vi "getPieces.vi"(0 "Refnum in":T1, 5 "Bounding Box":cluster{"x":sgl, "y":sgl}[][](array[cluster]), 7 "Position":sgl[][](array[numeric]), 9 "Angle":sgl[](array[numeric]), 11 "error in (no error)":errorcluster, 12 "Step":sgl=0.29742944, 13 "Origin Pixel":dbl[](array[numeric])) -> (4 "Refnum out":T1, 8 "Data Pieces":T3(array[cluster]) {"ROI Números"."Contours"."Type" items=["No Selection", "Point", "Line", "Rectangle", "Oval", "Polygon", "Freehand Region", "Annulus", "Unused2", "Unused3", "Broken Line", "Freehand Line", "Rotated Rectangle"]}, 15 "error out":errorcluster)   [LabVIEW 2016]
uses:
  <vilib>/vision/Image Controls.llb/IMAQ Image.ctl
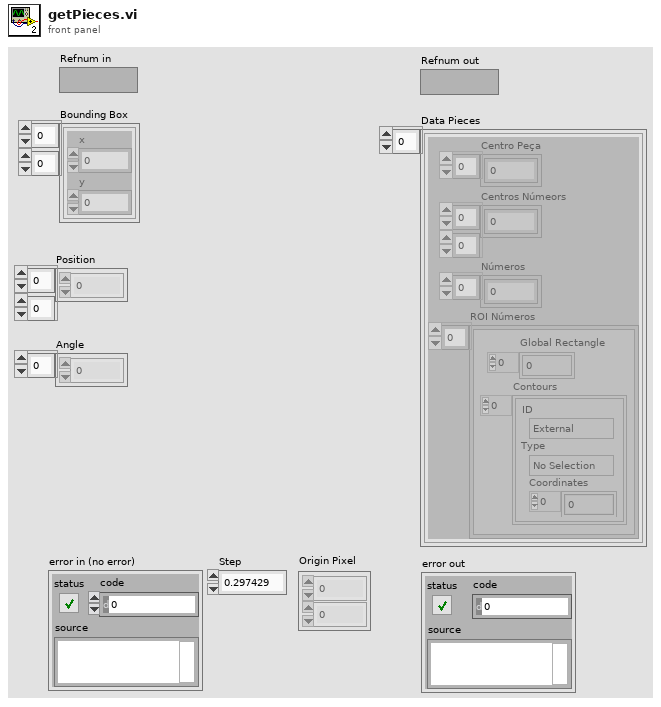
[diagram p1: front panel]
types:
  T1 = typedef "IMAQ Image.ctl" = refnum<image>
  T2 = typedef "ROI Descriptor" = cluster{"Global Rectangle":i32[], "Contours":cluster{"ID":enum32{"External", "Internal"}, "Type":u32, "Coordinates":i32[]}[]}
  T3 = cluster{"Centro Peça":dbl[], "Centros Númeors":dbl[][], "Números":u8[], "ROI Números":T2[]}[]
  T4 = cluster{"Centro Peça":dbl[], "Centros Númeors":dbl[][], "Números":u8[], "ROI Números":T2[]}
  T5 = typedef "IMAQ Rectangle" = cluster{"Left":i32, "Top":i32, "Right":i32, "Bottom":i32, "Rotation":dbl}
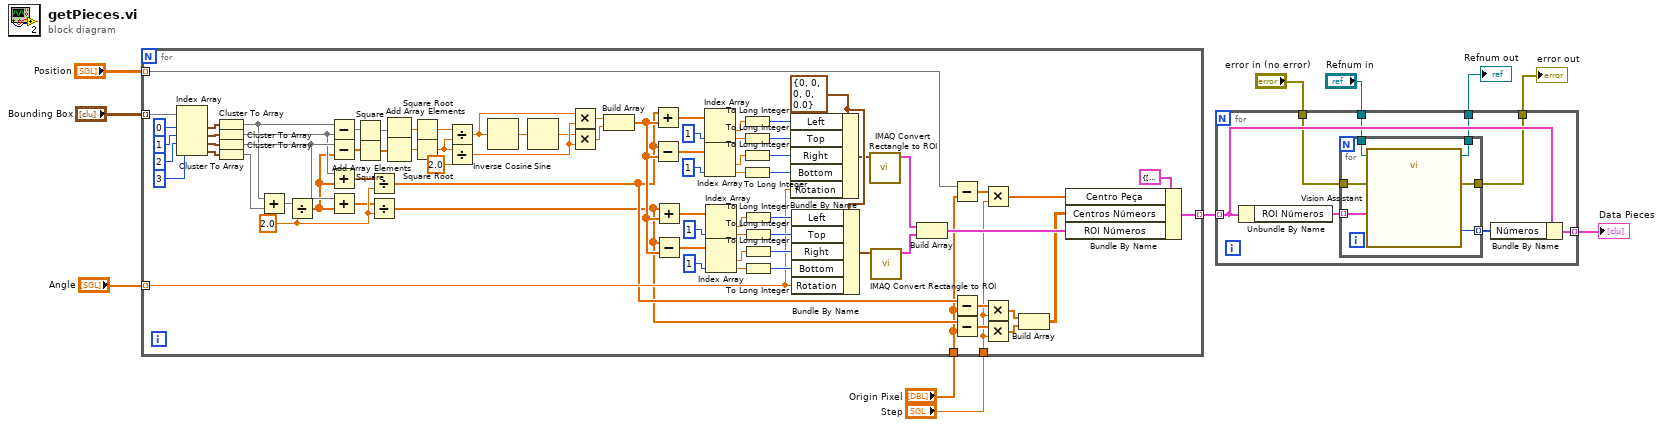
[diagram p0: block diagram]
diagram:
  n1 = for {
    tunnel: "Angle" -> [w29] mode=indexing
    tunnel: "Position" -> [w18] mode=indexing
    tunnel: "Bounding Box" -> [w30] mode=indexing
    tunnel: [w28] -> w4 mode=indexing
    tunnel: "Origin Pixel" -> [w13]
    tunnel: "Step" -> [w12]
    w89 = T5 {"Left"=0, "Top"=0, "Right"=0, "Bottom"=0, "Rotation"=0.0} ("Rectangle")
    w53 = 2.0 ("y")
    n2 = Index Array(array=w30, index #1=0 ("index"), index #2=1 ("index"), index #3=2 ("index"), index #4=3 ("index")) -> (element #1=w35:cluster{"x":sgl, "y":sgl}, element #2=w36:cluster{"x":sgl, "y":sgl}, element #3=w37:cluster{"x":sgl, "y":sgl}, element #4=w38:cluster{"x":sgl, "y":sgl})
    n3 = Cluster To Array(cluster=w35) -> (array=w47:sgl[])
    n4 = Cluster To Array(cluster=w36) -> (array=w49:sgl[])
    n5 = Cluster To Array(cluster=w37) -> (array=w50:sgl[])
    n6 = Cluster To Array(cluster=w38) -> (array=w42:sgl[])
    n7 = Add(x=w47, y=w42) -> (x+y=w43:sgl[])
    n8 = Divide(x=w43, y=w53) -> (x/y=w48:dbl[])
    n9 = Subtract(x=w47, y=w49) -> (x-y=w46:sgl[])
    n10 = Subtract(x=w50, y=w48) -> (x-y=w41:dbl[])
    n11 = Add(x=w49, y=w48) -> (x+y=w51:dbl[])
    n12 = Add(x=w50, y=w48) -> (x+y=w52:dbl[])
    n13 = Square(x=w46) -> (x^2=w44:sgl[])
    n14 = Square(x=w41) -> (x^2=w39:dbl[])
    n15 = Divide(x=w51, y=w53) -> (x/y=w23:dbl[])
    n16 = Divide(x=w52, y=w53) -> (x/y=w22:dbl[])
    n17 = Add Array Elements(numeric array=w44) -> (sum=w45:sgl)
    n18 = Add Array Elements(numeric array=w39) -> (sum=w40:dbl)
    n19 = Square Root(x=w45) -> (sqrt(x)=w54:sgl)
    n20 = Square Root(x=w40) -> (sqrt(x)=w55:dbl)
    n21 = Divide(x=w54, y=w55) -> (x/y=w61:dbl)
    n22 = Divide(x=w55, y=2.0) -> (x/y=w62:dbl)
    n23 = Inverse Cosine(1:w61) -> (0:w57:dbl)
    n24 = Sine(x=w57) -> (sin(x)=w58:dbl)
    n25 = Multiply(x=w61, y=w62) -> (x*y=w60:dbl)
    n26 = Multiply(x=w58, y=w62) -> (x*y=w59:dbl)
    n27 = Build Array(w60, w59) -> (w90:dbl[])
    n28 = Add(x=w23, y=w90) -> (x+y=w75:dbl[])
    n29 = Subtract(x=w23, y=w90) -> (x-y=w74:dbl[])
    n30 = Add(x=w22, y=w90) -> (x+y=w88:dbl[])
    n31 = Subtract(x=w22, y=w90) -> (x-y=w87:dbl[])
    n32 = Index Array(array=w75, index #2=1 ("index")) -> (element #1=w73:dbl, element #2=w72:dbl)  [unwired: 1 in]
    n33 = Index Array(array=w74, index #2=1 ("index")) -> (element #1=w71:dbl, element #2=w70:dbl)  [unwired: 1 in]
    n34 = Index Array(array=w88, index #2=1 ("index")) -> (element #1=w86:dbl, element #2=w85:dbl)  [unwired: 1 in]
    n35 = Index Array(array=w87, index #2=1 ("index")) -> (element #1=w84:dbl, element #2=w83:dbl)  [unwired: 1 in]
    n36 = To Long Integer(number=w73) -> (32bit integer=w66:i32)
    n37 = To Long Integer(number=w72) -> (32bit integer=w67:i32)
    n38 = To Long Integer(number=w71) -> (32bit integer=w68:i32)
    n39 = To Long Integer(number=w70) -> (32bit integer=w69:i32)
    n40 = To Long Integer(number=w86) -> (32bit integer=w79:i32)
    n41 = To Long Integer(number=w85) -> (32bit integer=w80:i32)
    n42 = To Long Integer(number=w84) -> (32bit integer=w81:i32)
    n43 = To Long Integer(number=w83) -> (32bit integer=w82:i32)
    n44 = Bundle By Name(cluster=w89, "Left"=w66, "Top"=w67, "Right"=w68, "Bottom"=w69, "Rotation"=w29) -> (w65:T5)
    n45 = Bundle By Name(cluster=w89, "Left"=w79, "Top"=w80, "Right"=w81, "Bottom"=w82, "Rotation"=w29) -> (w78:T5)
    n46 = call "IMAQ Convert Rectangle to ROI"("Rectangle"=w65) -> ("ROI Descriptor"=w26:T2)  [unwired: 8 in, 1 out]
    n47 = call "IMAQ Convert Rectangle to ROI"("Rectangle"=w78) -> ("ROI Descriptor"=w25:T2)  [unwired: 8 in, 1 out]
    n48 = Build Array(w26, w25) -> (w24:T2[])
    n49 = Subtract(x=w18, y=w13) -> (x-y=w19:dbl[])
    n50 = Subtract(x=w23, y=w13) -> (x-y=w21:dbl[])
    n51 = Subtract(x=w22, y=w13) -> (x-y=w20:dbl[])
    n52 = Multiply(x=w19, y=w12) -> (x*y=w17:dbl[])
    n53 = Multiply(x=w21, y=w12) -> (x*y=w16:dbl[])
    n54 = Multiply(x=w20, y=w12) -> (x*y=w15:dbl[])
    n55 = Build Array(w16, w15) -> (w14:dbl[][])
    n56 = Bundle By Name(cluster=T4 {"Centro Peça"=[0.0, 0.0], "Centros Númeors"=[[0.0, 0.0], [0.0, 0.0]], "Números"=[0, 0], "ROI Números"=[]} ("Dados Peça"), "Centro Peça"=w17, "Centros Númeors"=w14, "ROI Números"=w24) -> (w28:T4)
  }
  n57 = for {
    tunnel: w4 -> [w98] mode=indexing
    tunnel: [w97] -> w5 mode=indexing
    tunnel: "error in (no error)" -> [w96]
    tunnel: [w95] -> w10
    tunnel: "Refnum in" -> [w94]
    tunnel: [w91] -> w3
    n58 = Unbundle By Name(w98) -> ("ROI Números"=w93:T2[])
    n59 = for {
      tunnel: w94 -> [w102]
      tunnel: w96 -> [w104]
      tunnel: [w103] -> w95
      tunnel: w93 -> [w101] mode=indexing
      tunnel: [w100] -> w92 mode=indexing
      tunnel: [w99] -> w91
      n60 = call "Vision Assistant"("Image In"=w102, "ROI Descriptor (Image Mask 1)"=w101, "error in"=w104) -> ("Image Out"=w99:T1, "Number of Particles (Particle Analysis 1)"=w100:i32, "error out"=w103:errorcluster)  [unwired: 22 in]
    }
    n61 = Bundle By Name(cluster=w98, "Números"=w92) -> (w97:T4)
  }
  "error out" <- w10
  "Data Pieces" <- w5
  "Refnum out" <- w3
